vi "Log Error.vi"(8 "error in (no error)":errorcluster, 10 "Error Data":T1, 11 "ATM Controller in":refnum<class "ATM Controller.lvclass">) -> (0 "error out":errorcluster, 3 "ATM Controller out":refnum<class "ATM Controller.lvclass">)   [LabVIEW 2019, in "ATM Controller.lvlib" / "ATM Controller.lvclass"]
uses:
  ATM Controller.lvclass
  Error Level.ctl
  Error Data.ctl
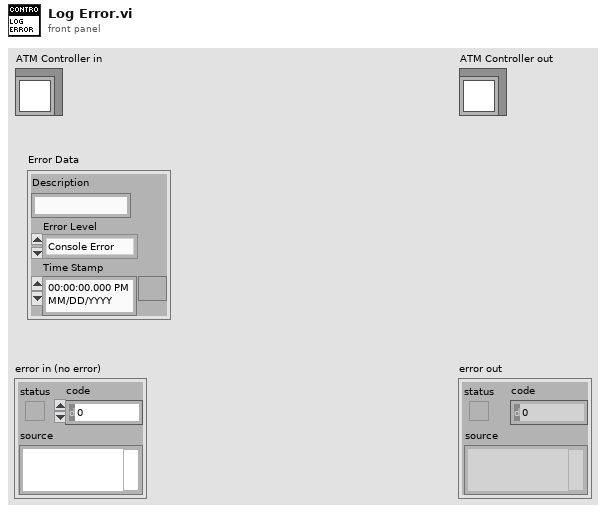
[diagram p1: front panel]
types:
  T1 = typedef "ATM Controller.lvlib/ATM Controller.lvclass/Error Data.ctl" = cluster{"Description":string, "Error Level":T2, "Time Stamp":timestamp}
  T2 = typedef "ATM Controller.lvlib/ATM Controller.lvclass/Error Level.ctl" = enum16{"Console Error", "Sensor Interface IO Error", "Process Step Error"}
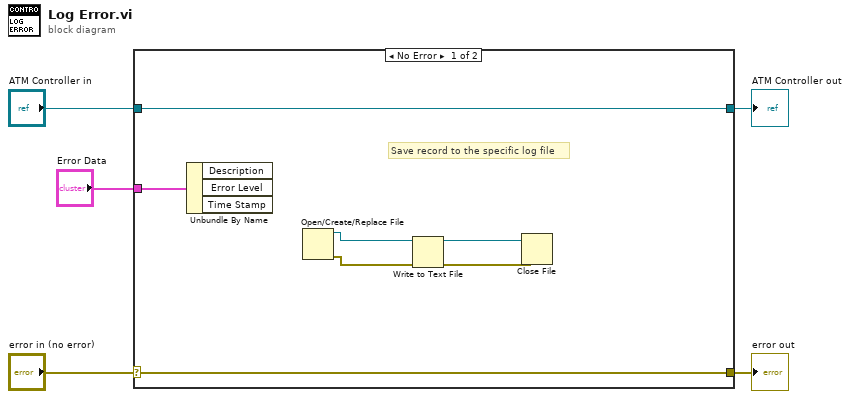
[diagram p0: block diagram]
diagram:
  n1 = case shown="No Error" "error in (no error)" {
    selector: "error in (no error)" -> [w11 w14]
    tunnel: [w11 w14] -> w4
    tunnel: [w12 w13] -> w2
    tunnel: "ATM Controller in" -> [w12 w13]
    tunnel: "Error Data" -> [w6 _]
    frame No Error {
      # "Save record to the specific log file"
      n2 = Unbundle By Name(w6) -> ()  [unwired: 3 out]
      n3 = Open/Create/Replace File() -> (refnum out=w8:refnum<file>, error out=w10:errorcluster)  [unwired: 6 in, 1 out]
      n4 = Write to Text File(file (use dialog)=w8, error in=w10) -> (refnum out=w7:refnum<file>, error out=w9:errorcluster)  [unwired: 2 in, 1 out]
      n5 = Close File(refnum=w7, error in=w9) -> ()  [unwired: 2 out]
    }
    frame Error {
    }
  }
  "error out" <- w4
  "ATM Controller out" <- w2
